vi "Monitor Time.vi"(8 "error in (no error)":errorcluster, 10 "Address (0)":i32, 11 "VISA resource name":refnum<visa-resource-name>) -> (0 "error out":errorcluster, 1 "Second":i32, 2 "Minute":i32, 3 "VISA resource name out":refnum<visa-resource-name>, 4 "Time":dbl format="%<%H:%M:%S>t", 5 "Hour":i32)   [LabVIEW 2016, in "Environment Chamber.lvlib" / "Climatic Chamber.lvlib"]
doc: "<b>Time monitor</b>\n\nReturns the current time of the internal calendar."
uses:
  Climatic Chamber.lvlib
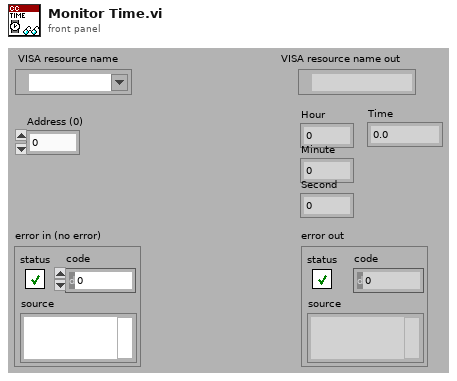
[diagram p1: front panel]
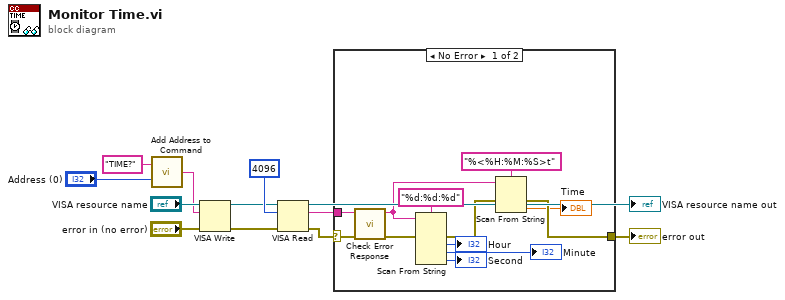
[diagram p0: block diagram]
diagram:
  n1 = call "Add Address to Command.vi"("Address (0)"="Address (0)", "Command"="TIME?") -> ("Command OUT"=w5:string)
  n2 = VISA Write(VISA resource name="VISA resource name", write buffer=w5, error in (no error)="error in (no error)") -> (VISA resource name out=w9:refnum<visa-resource-name>, error out=w8:errorcluster)  [unwired: 1 out]
  n3 = VISA Read(VISA resource name=w9, byte count=u32 4096, error in (no error)=w8) -> (VISA resource name out=→"VISA resource name out":refnum<visa-resource-name>, read buffer=w3:string, error out=w4:errorcluster)  [unwired: 1 out]
  n4 = case shown="No Error" w4 {
    selector: w4 -> [w22 w25]
    tunnel: w3 -> [w23 _]
    tunnel: [w24 w25] -> w2
    frame No Error {
      n5 = call "Check Error Response.vi"("error in (no error)"=w22, "read String"=w23) -> ("error out"=w21:errorcluster, "String out"=w16:string)  [unwired: 7 in, 1 out]
      n6 = Scan From String(format string="%d:%d:%d", input string=w16, error in=w21) -> (error out=w13:errorcluster, output 1=→"Hour":i32, output 2=→"Minute":i32, output 3=→"Second":i32)  [unwired: 4 in, 2 out]
      n7 = Scan From String(format string="%<%H:%M:%S>t", input string=w16, error in=w13) -> (error out=w24:errorcluster, output 1=→"Time":dbl)  [unwired: 2 in, 2 out]
    }
    frame Error {
    }
  }
  "error out" <- w2
